vi "test2.vi"() -> ()   [LabVIEW 2010]
uses:
  <vilib>/picture/3D Picture Control/NI_3D Picture Control.lvlib
panel:
  out "3D Picture":refnum<vi>(3d-picture)
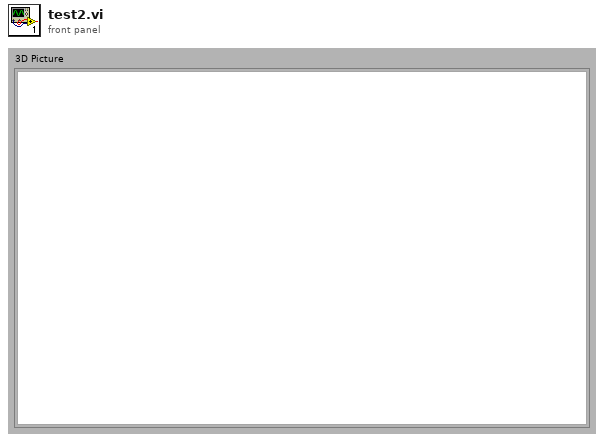
[diagram p1: front panel]
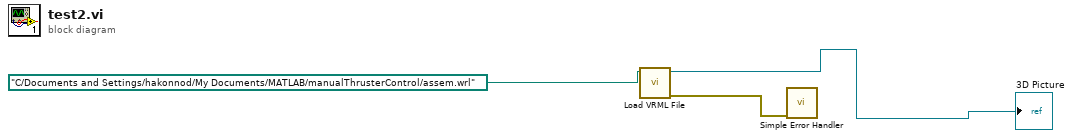
[diagram p0: block diagram]
diagram:
  n1 = call <vilib>:"Load VRML File.vi"("Path"=path "C:/Documents and Settings/hakonnod/My Documents/MATLAB/manualThrusterControl/assem.wrl") -> ("error out"=w2:errorcluster, "Scene:Read Scene File"=→"3D Picture":refnum<vi>)  [unwired: 9 in]
  n2 = call <vilib>:"Simple Error Handler.vi"("error in (no error)"=w2) -> ()  [unwired: 4 in, 5 out]
